vi "setFPGA.vi"(10 "FPGA":refnum<class "FPGA.lvclass">, 11 "ModbusSubnetATxDataFIFO in":refnum<class "ModbusSubnetATxDataFIFO.lvclass">) -> (3 "ModbusSubnetATxDataFIFO out":refnum<class "ModbusSubnetATxDataFIFO.lvclass">)   [LabVIEW 2016, in "ModbusSubnetATxDataFIFO.lvclass"]
uses:
  ModbusSubnetATxDataFIFO.lvclass
  FPGA/FPGA.lvclass
  ModbusSubnetATxDataFIFO.lvclass/ModbusSubnetATxDataFIFO.ctl
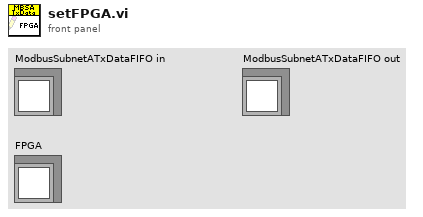
[diagram p1: front panel]
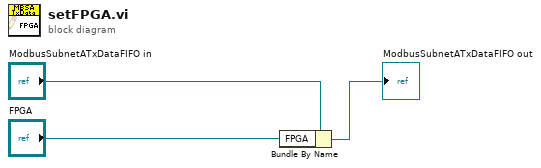
[diagram p0: block diagram]
diagram:
  n1 = Bundle By Name(cluster="ModbusSubnetATxDataFIFO in", "FPGA"="FPGA") -> (→"ModbusSubnetATxDataFIFO out":refnum<class "ModbusSubnetATxDataFIFO.lvclass">)
